vi "Process Beacon.vi"(0 "Known Hosts in":T1[](array[typedef]), 7 "DiscoveredHost":T1={"Beacon"={"name"="", "addr"="", "port"=0, "ver"=10001}, "Last Seen"=timestamp(0 s since 1904-01-01)}) -> (4 "Known Hosts out":T1[](array[typedef]), 8 "Beacon Result":T3)   [LabVIEW 2020]
uses:
  Public/Discovery/Typedefs/Beacon Result.ctl
  Discovered Host.ctl
  Public/Discovery/Typedefs/Server Beacon.ctl
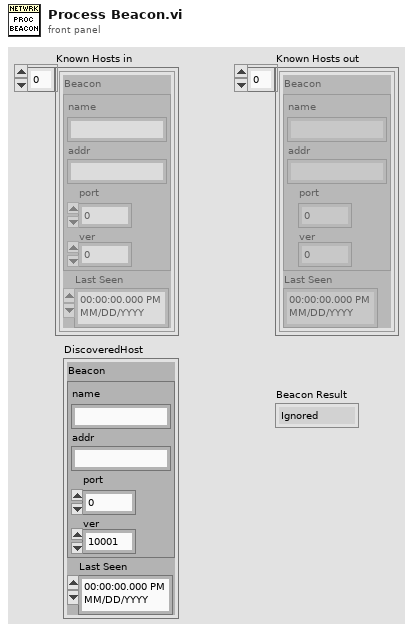
[diagram p1: front panel]
types:
  T1 = typedef "Discovered Host.ctl" = cluster{"Beacon":T2, "Last Seen":timestamp}
  T2 = typedef "Server Beacon.ctl" = cluster{"name":string, "addr":string, "port":u16, "ver":u16}
  T3 = typedef "Beacon Result.ctl" = enum16{"Ignored", "Updated", "Added"}
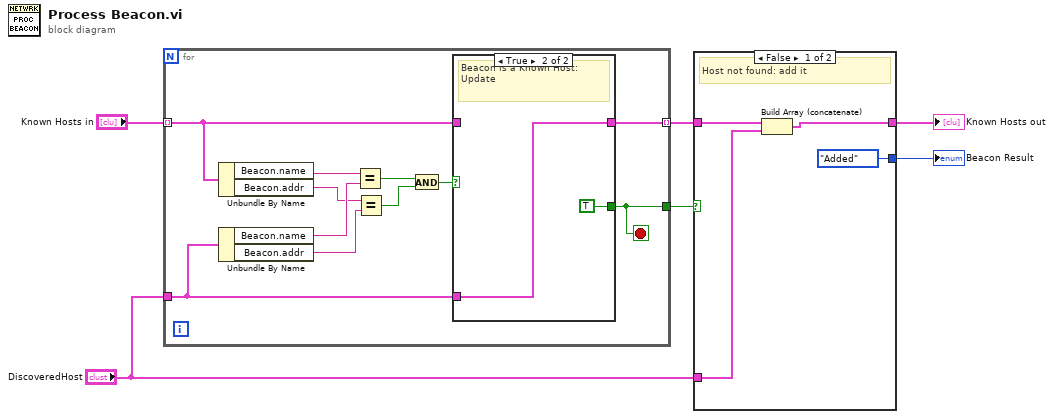
[diagram p0: block diagram]
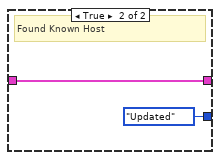
[diagram p2: hidden frame]
diagram:
  n1 = for {
    tunnel: "Known Hosts in" -> [w13] mode=indexing
    tunnel: "DiscoveredHost" -> [w12]
    tunnel: [w11] -> w4 mode=indexing
    tunnel: [w10] -> w5
    stop <- w10 stop-if-true
    n2 = Unbundle By Name(w13) -> ("Beacon.name"=w17:string, "Beacon.addr"=w15:string)
    n3 = Unbundle By Name(w12) -> ("Beacon.name"=w16:string, "Beacon.addr"=w14:string)
    n4 = Equal?(x=w17, y=w16) -> (x = y?=w9:bool)
    n5 = Equal?(x=w15, y=w14) -> (x = y?=w8:bool)
    n6 = And(x=w9, y=w8) -> (x .and. y?=w7:bool)
    n7 = case shown="True" w7 {
      tunnel: w13 -> [w18 _]
      tunnel: w12 -> [_ w19]
      tunnel: [w18 w19] -> w11
      tunnel: [_ TRUE] -> w10
      frame False {
      }
      frame True {
        # "Beacon is a Known Host:\nUpdate"
      }
    }
  }
  n8 = case shown="False" w5 {
    tunnel: w4 -> [w24 w26]
    tunnel: [w22 w26] -> w2
    tunnel: "DiscoveredHost" -> [w23 _]
    tunnel: [Beacon_Result."Added" ("Beacon Result") Beacon_Result."Updated" ("Beacon Result")] -> w1
    frame False {
      # "Host not found: add it"
      n9 = Build Array (concatenate)(w24, w23) -> (w22:T1[])
    }
    frame True {
      # "Found Known Host"
    }
  }
  "Beacon Result" <- w1
  "Known Hosts out" <- w2
